vi "User Dynamic (single).vi"(7 "User.lvclass":refnum<class "User.lvclass">, 8 "error in (no error)":errorcluster, 11 "XY-data":cluster{"X-array":dbl[], "Y-array":dbl[]} {"Y-array" format="%.2p"; "X-array" format="%.2p"}) -> (0 "error out":errorcluster, 3 "XY-data out":cluster{"X-array":dbl[], "Y-array":dbl[]} {"Y-array" format="%.2p"; "X-array" format="%.2p"}, 5 "User.lvclass out":refnum<class "User.lvclass">)   [LabVIEW 2019, in "User.lvclass"]
uses:
  User.lvclass
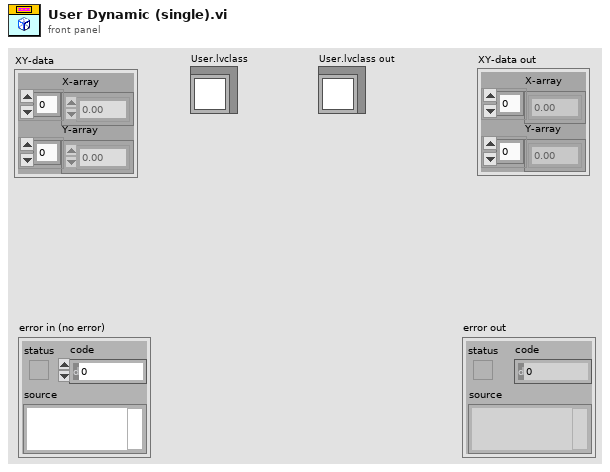
[diagram p1: front panel]
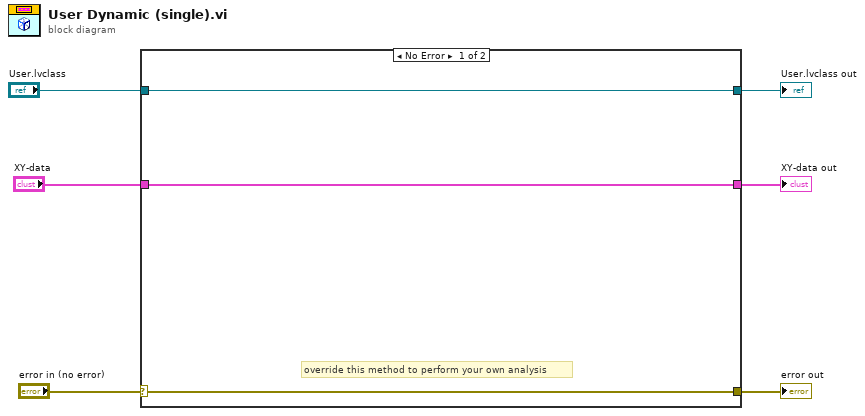
[diagram p0: block diagram]
diagram:
  n1 = case shown="No Error" "error in (no error)" {
    selector: "error in (no error)" -> [w9 w12]
    tunnel: [w9 w12] -> w5
    tunnel: "XY-data" -> [w8 w11]
    tunnel: [w8 w11] -> w3
    tunnel: [w7 w10] -> w1
    tunnel: "User.lvclass" -> [w7 w10]
    frame No Error {
      # "override this method to perform your own analysis"
    }
    frame Error {
    }
  }
  "error out" <- w5
  "XY-data out" <- w3
  "User.lvclass out" <- w1
